vi "PhotonPipelineMetadata_Unpack.vi"(11 "RawData":u8[](array[numeric])) -> (1 "NextByte":i32, 3 "PhotonPipelineMetadata":T1)   [LabVIEW 2019, in "PhotonVisionLib.lvlib"]
doc: "Internal function to parse the data returned by PhotonCamera_GetLatestResult.\n\nInputs:\n - RawData -- Byte array containing the data to parse.\n\nOutputs:\n - PipelineMetadata -- Parsed PipelineMetadata cluster."
uses:
  PhotonVisionLib.lvlib
  TypeDef/PhotonPipelineMetadataType.ctl
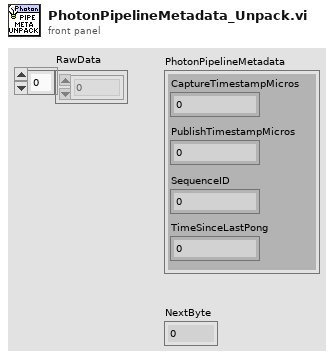
[diagram p1: front panel]
types:
  T1 = typedef "PhotonVisionLib.lvlib/PhotonPipelineMetadataType.ctl" = cluster{"CaptureTimestampMicros":i64, "PublishTimestampMicros":i64, "SequenceID":i64, "TimeSinceLastPong":i64}
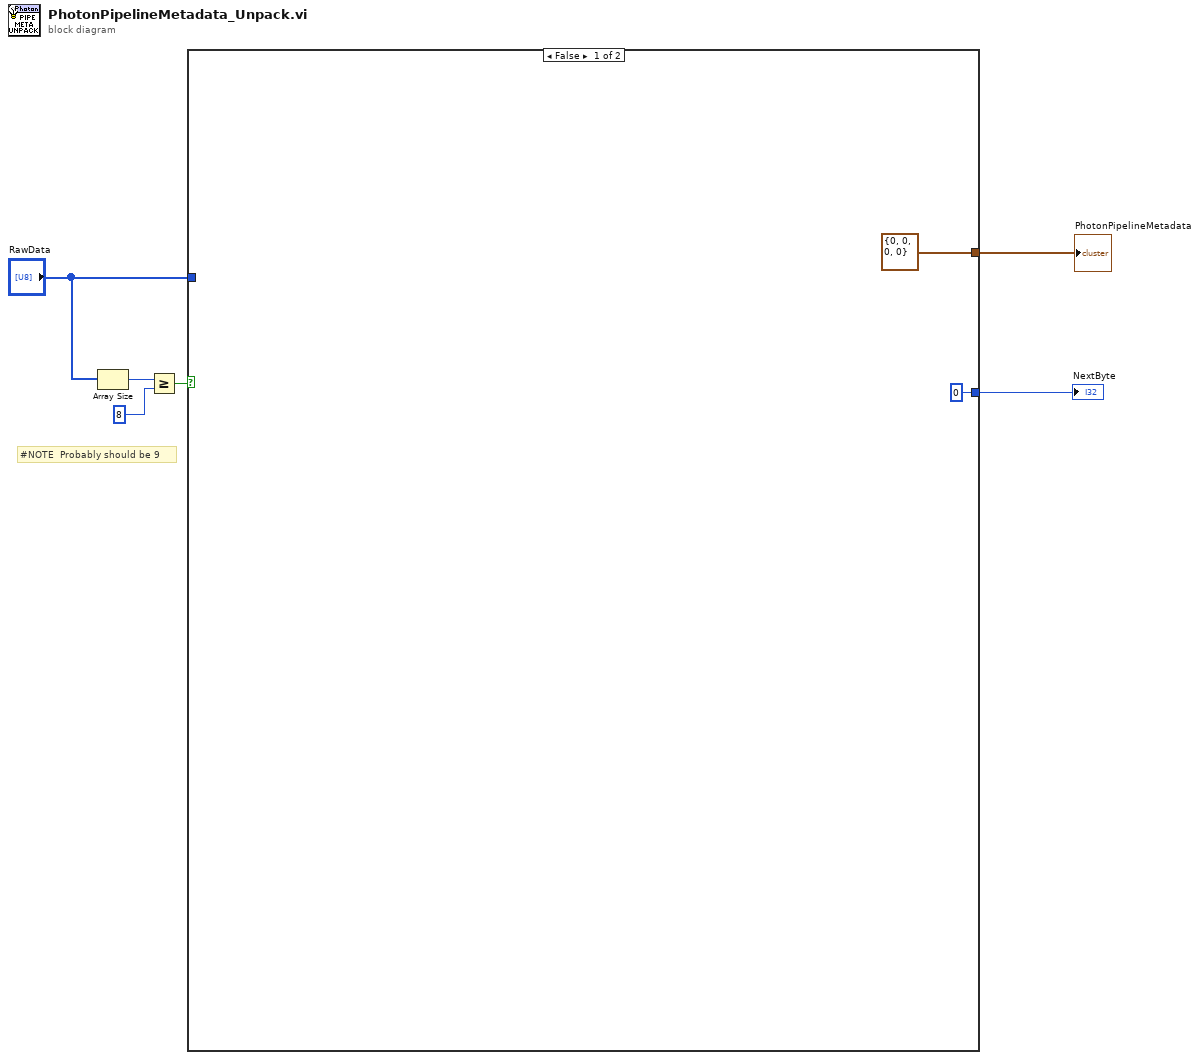
[diagram p0: block diagram]
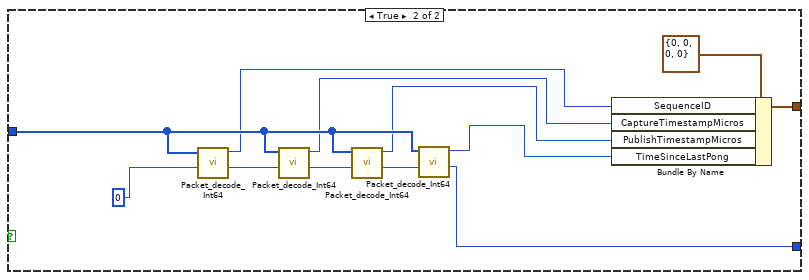
[diagram p2: hidden frame]
diagram:
  # "#NOTE  Probably should be 9"
  n1 = Array Size(array="RawData") -> (size(s)=w5:i32)
  n2 = Greater Or Equal?(x=w5, y=8) -> (x >= y?=w6:bool)
  n3 = case shown="False" w6 {
    tunnel: "RawData" -> [_ w14]
    tunnel: [T1 {"CaptureTimestampMicros"=0, "PublishTimestampMicros"=0, "SequenceID"=0, "TimeSinceLastPong"=0} ("PhotonPipelineMetadata") w18] -> w2
    tunnel: [0 ("NextByte") w9] -> w1
    frame False {
    }
    frame True {
      n4 = call "Packet_decode_Int64.vi"("StartByte"=0, "RawData"=w14) -> ("NextByte"=w17:i32, "Int64_Value"=w13:i64)  [unwired: 8 in]
      n5 = call "Packet_decode_Int64.vi"("StartByte"=w17, "RawData"=w14) -> ("NextByte"=w16:i32, "Int64_Value"=w12:i64)  [unwired: 8 in]
      n6 = call "Packet_decode_Int64.vi"("StartByte"=w16, "RawData"=w14) -> ("NextByte"=w15:i32, "Int64_Value"=w11:i64)  [unwired: 8 in]
      n7 = call "Packet_decode_Int64.vi"("StartByte"=w15, "RawData"=w14) -> ("NextByte"=w9:i32, "Int64_Value"=w10:i64)  [unwired: 8 in]
      n8 = Bundle By Name(cluster=T1 {"CaptureTimestampMicros"=0, "PublishTimestampMicros"=0, "SequenceID"=0, "TimeSinceLastPong"=0} ("PhotonPipelineMetadata"), "SequenceID"=w13, "CaptureTimestampMicros"=w12, "PublishTimestampMicros"=w11, "TimeSinceLastPong"=w10) -> (w18:T1)
    }
  }
  "PhotonPipelineMetadata" <- w2
  "NextByte" <- w1
